vi "make_subvi_metaarray.vi"(10 "UID":string, 11 "VIPath":path) -> (3 "数组":string[](array[string]))   [LabVIEW 2020]
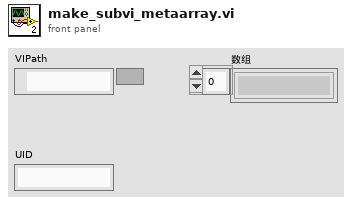
[diagram p1: front panel]
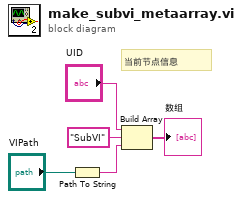
[diagram p0: block diagram]
diagram:
  # "当前节点信息"
  n1 = Path To String(path="VIPath") -> (string=w2:string)
  n2 = Build Array("UID", "SubVI" ("y"), w2) -> (→"数组":string[])
